vi "time delay.vi"(8 "error in (no error)":errorcluster, 11 "timer delay (s)":dbl=5.0 format="%.4g") -> (0 "error out":errorcluster, 2 "done?":bool=TRUE)   [LabVIEW 2020]
panel:
  out "ms to go":u32
  out "timer (ms)":u32
  out "target (ms)":dbl
  out "timer start (ms)":u32
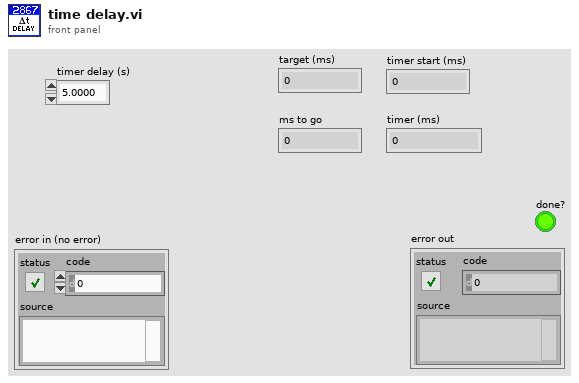
[diagram p1: front panel]
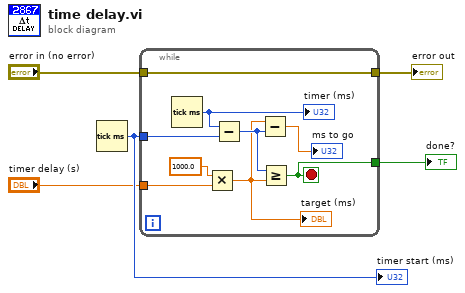
[diagram p0: block diagram]
diagram:
  n1 = Tick Count (ms)() -> (millisecond timer value=w5:u32)
  "timer start (ms)" <- w5
  n2 = while {
    tunnel: w5 -> [w11]
    tunnel: "timer delay (s)" -> [w14]
    tunnel: [w9] -> w2
    tunnel: "error in (no error)" -> [w9]
    tunnel: [w6] -> w1
    stop <- w6 stop-if-true
    n3 = Tick Count (ms)() -> (millisecond timer value=w12:u32)
    "timer (ms)" <- w12
    n4 = Multiply(x=1000.0, y=w14) -> (x*y=w7:dbl)
    "target (ms)" <- w7
    n5 = Subtract(x=w12, y=w11) -> (x-y=w10:u32)
    n6 = Subtract(x=w7, y=w10) -> (x-y=→"ms to go":dbl)
    n7 = Greater Or Equal?(x=w10, y=w7) -> (x >= y?=w6:bool)
  }
  "error out" <- w2
  "done?" <- w1
